vi "Stop Test.vi"(8 "error in (no error)":errorcluster, 11 "XML Report in":refnum<class "Report.lvclass">) -> (0 "error out":errorcluster, 3 "XML Report out":refnum<class "Report.lvclass">)   [LabVIEW 2020, in "Reports.lvlib" / "Report.lvclass"]
uses:
  Report.lvclass
  Report.lvclass/Report.ctl
  Report Generator/Report Generator.lvclass
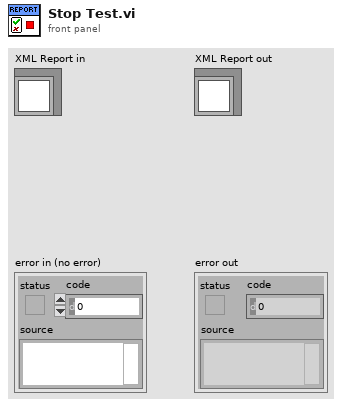
[diagram p1: front panel]
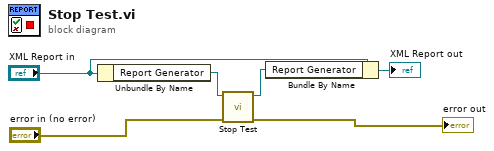
[diagram p0: block diagram]
diagram:
  n1 = Unbundle By Name("XML Report in") -> ("Report Generator"=w5:refnum<class "Report Generator.lvclass">)
  n2 = call "Stop Test.vi"("error in (no error)"="error in (no error)", "Report Generator In"=w5) -> ("error out"=→"error out":errorcluster, "Report Generator Out"=w3:refnum<class "Report Generator.lvclass">)  [unwired: 8 in]
  n3 = Bundle By Name(cluster="XML Report in", "Report Generator"=w3) -> (→"XML Report out":refnum<class "Report.lvclass">)
